vi "MorseCode_Project.vi"() -> ()   [LabVIEW 2012]
panel:
  in  "Stop":bool
  in  "Clear":bool
  in  "Decode":bool
  out "Decoded Text":string
  in  "Morse input":string
  in  "Encode":bool
  out "Morse Output":string
  in  "Text Input":string
  # "Encoder Section"
  # "Ayush Jangra\n2410994514"
  # "Decoder Section"
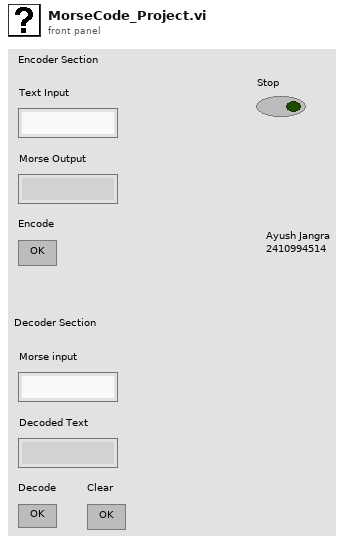
[diagram p1: front panel]
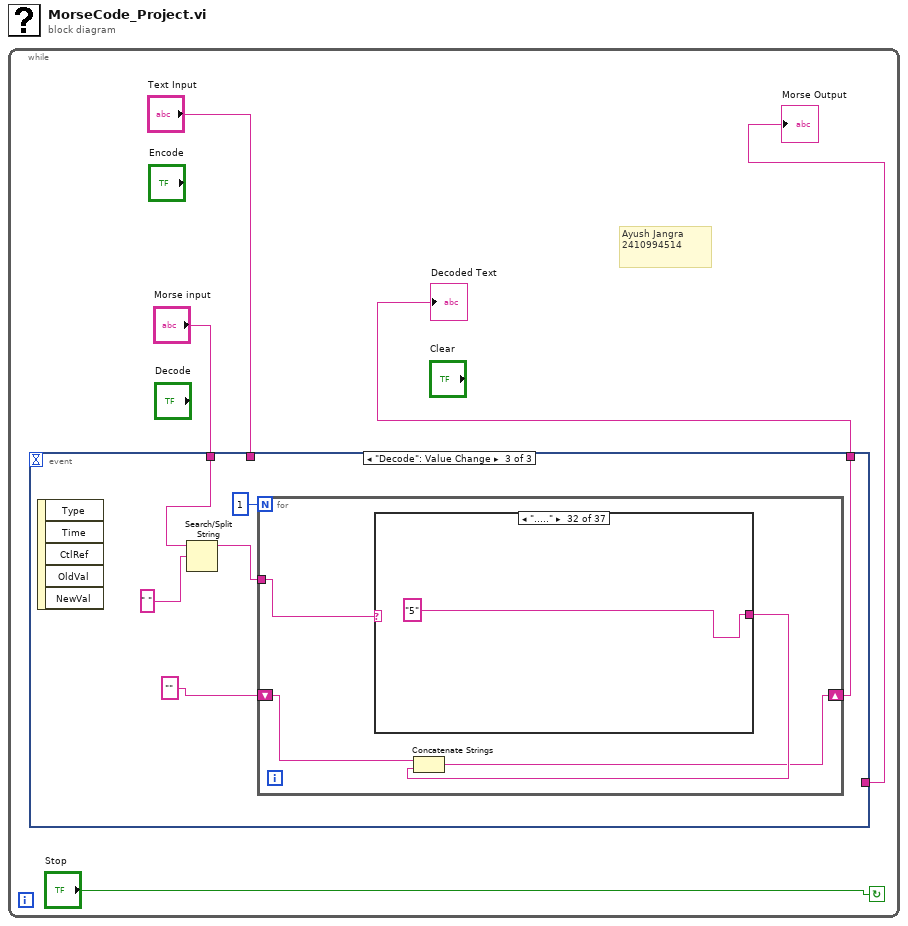
[diagram p0: block diagram]
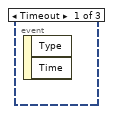
[diagram p2: hidden frame]
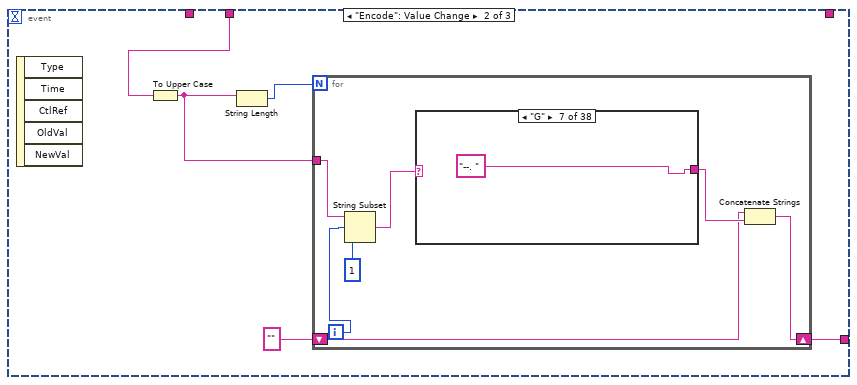
[diagram p3: hidden frame]
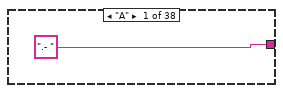
[diagram p4: hidden frame]
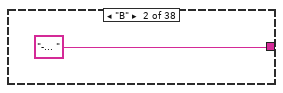
[diagram p5: hidden frame]
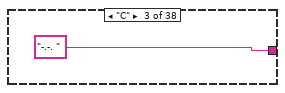
[diagram p6: hidden frame]
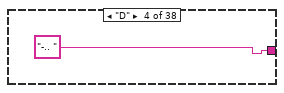
[diagram p7: hidden frame]
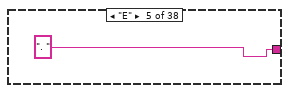
[diagram p8: hidden frame]
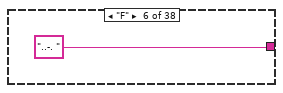
[diagram p9: hidden frame]
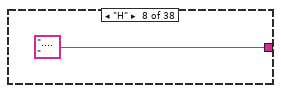
[diagram p10: hidden frame]
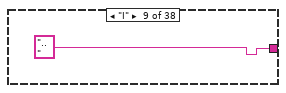
[diagram p11: hidden frame]
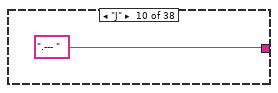
[diagram p12: hidden frame]
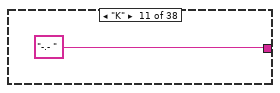
[diagram p13: hidden frame]
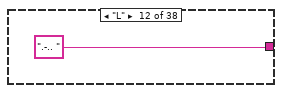
[diagram p14: hidden frame]
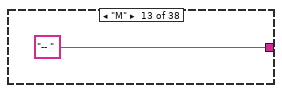
[diagram p15: hidden frame]
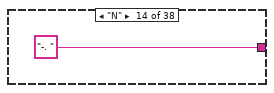
[diagram p16: hidden frame]
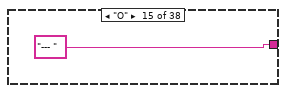
[diagram p17: hidden frame]
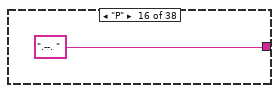
[diagram p18: hidden frame]
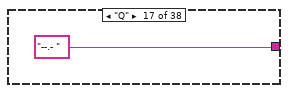
[diagram p19: hidden frame]
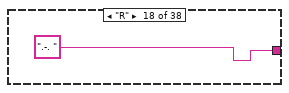
[diagram p20: hidden frame]
diagram:
  n1 = while {
    stop <- "Stop" continue-if-true
    # "Ayush Jangra\n2410994514"
    n2 = event shown="[2] \"Decode\": Value Change" {
      selector: _ -> [_ _ _]
      dyn-events: _ -> [_ _ _]
      timeout: _ -> [_ _ _]
      tunnel: "Text Input" -> [_ w10 _]
      tunnel: [_ w6 _] -> w3
      tunnel: "Morse input" -> [_ _ w60]
      tunnel: [_ _ w57] -> w1
      event Timeout {
        n3 = event-data() -> ()  [unwired: 1 in, 2 out]
      }
      event "Encode": Value Change {
        n4 = event-data() -> ()  [unwired: 1 in, 5 out]
        n5 = To Upper Case(1:w10) -> (0:w8:string)
        n6 = String Length(string=w8) -> (length=w9:i32)
        n7 = for {
          N: w9 -> [_]
          tunnel: w8 -> [w14]
          shift-right: [w15] -> w6
          shift-left: "" -> [w16]
          i -> [w13]
          n8 = String Subset(string=w14, offset (0)=w13, length (rest)=1 ("length (rest)")) -> (substring=w11:string)
          n9 = case shown="\"G\"" w11 {
            tunnel: [".- " "-... " "-.-. " "-.. " ". " "..-. " "--. " ".... " ".. " ".--- " "-.- " ".-.. " "-- " "-. " "--- " ".--. " "--.- " ".-. " "... " "- " "..- " "...- " ".-- " "-..- " "-.-- " "--.. " "----- " ".---- " "..--- " "...-- " "....- " "..... " "-.... " "--... " "---.. " "----. " " / " _] -> w17
            frame "A" {
            }
            frame "B" {
            }
            frame "C" {
            }
            frame "D" {
            }
            frame "E" {
            }
            frame "F" {
            }
            frame "G" {
            }
            frame "H" {
            }
            frame "I" {
            }
            frame "J" {
            }
            frame "K" {
            }
            frame "L" {
            }
            frame "M" {
            }
            frame "N" {
            }
            frame "O" {
            }
            frame "P" {
            }
            frame "Q" {
            }
            frame "R" {
            }
            frame "S" {
            }
            frame "T" {
            }
            frame "U" {
            }
            frame "V" {
            }
            frame "W" {
            }
            frame "X" {
            }
            frame "Y" {
            }
            frame "Z" {
            }
            frame "0" {
            }
            frame "1" {
            }
            frame "2" {
            }
            frame "3" {
            }
            frame "4" {
            }
            frame "5" {
            }
            frame "6" {
            }
            frame "7" {
            }
            frame "8" {
            }
            frame "9" {
            }
            frame " " {
            }
            frame Default {
            }
          }
          n10 = Concatenate Strings(w16, w17) -> (w15:string)
        }
      }
      event "Decode": Value Change {
        n11 = event-data() -> ()  [unwired: 1 in, 5 out]
        n12 = Search/Split String(string=w60, search string/char (-)=" ") -> (substring before match=w56:string)  [unwired: 1 in, 2 out]
        n13 = for {
          N: 1 -> [_]
          shift-right: [w62] -> w57
          shift-left: "" -> [w63]
          tunnel: w56 -> [w61]
          n14 = case shown="\".....\"" w61 {
            tunnel: ["A" "B" "C" "D" "E" "F" "G" "H" "I" "J" "K" "L" "M" "N" "O" "P" "Q" "R" "S" "T" "U" "V" "W" "X" "Y" "Z" "0" "1" "2" "3" "4" "5" "6" "7" "8" "9" "?"] -> w64
            frame ".-" {
            }
            frame "-..." {
            }
            frame "-.-." {
            }
            frame "-.." {
            }
            frame "." {
            }
            frame "..-." {
            }
            frame "--." {
            }
            frame "...." {
            }
            frame ".." {
            }
            frame ".---" {
            }
            frame "-.-" {
            }
            frame ".-.." {
            }
            frame "--" {
            }
            frame "-." {
            }
            frame "---" {
            }
            frame ".--." {
            }
            frame "--.-" {
            }
            frame ".-." {
            }
            frame "..." {
            }
            frame "-" {
            }
            frame "..-" {
            }
            frame "...-" {
            }
            frame ".--" {
            }
            frame "-..-" {
            }
            frame "-.--" {
            }
            frame "--.." {
            }
            frame "-----" {
            }
            frame ".----" {
            }
            frame "..---" {
            }
            frame "...--" {
            }
            frame "....-" {
            }
            frame "....." {
            }
            frame "-...." {
            }
            frame "--..." {
            }
            frame "---.." {
            }
            frame "----." {
            }
            frame Default {
            }
          }
          n15 = Concatenate Strings(w63, w64) -> (w62:string)
        }
      }
    }
    "Morse Output" <- w3
    "Decoded Text" <- w1
  }
